vi "KH7008 Parse Response String.vi"(8 "error in (no error)":errorcluster, 11 "Response String":string) -> (0 "error out":errorcluster, 3 "Channel Parameters":T1)   [LabVIEW 2019, in "Inst.Krohn-Hite-7008.lvclass"]
uses:
  Inst.Krohn-Hite-7008.lvclass
  Typedefs/SetAll-Cluster.ctl
  Typedefs/Channel-Enum.ctl
  Typedefs/Gain-Enum.ctl
  Typedefs/Filter-Enum.ctl
  Typedefs/Shunt-Enum.ctl
  Typedefs/Coupling-Enum.ctl
  Typedefs/Input Configuration-Enum.ctl
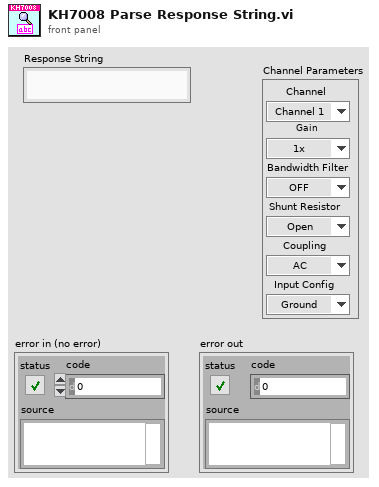
[diagram p1: front panel]
types:
  T1 = typedef "Inst.Krohn-Hite-7008.lvclass/SetAll-Cluster.ctl" = cluster{"Channel":T2, "Gain":T3, "Bandwidth Filter":T4, "Shunt Resistor":T5, "Coupling":T6, "Input Config":T7}
  T2 = typedef "Inst.Krohn-Hite-7008.lvclass/Channel-Enum.ctl" = enum16{"Channel 1", "Channel 2", "Channel 3", "Channel 4", "Channel 5", "Channel 6", "Channel 7", "Channel 8"}
  T3 = typedef "Inst.Krohn-Hite-7008.lvclass/Gain-Enum.ctl" = enum16{"1x", "10x", "100x", "1000x"}
  T4 = typedef "Inst.Krohn-Hite-7008.lvclass/Filter-Enum.ctl" = enum16{"OFF", "ON"}
  T5 = typedef "Inst.Krohn-Hite-7008.lvclass/Shunt-Enum.ctl" = enum16{"Open", "50 Ohms", "500 Ohms", "5k Ohms", "50k Ohms", "10M Ohm"}
  T6 = typedef "Inst.Krohn-Hite-7008.lvclass/Coupling-Enum.ctl" = enum16{"AC", "DC"}
  T7 = typedef "Inst.Krohn-Hite-7008.lvclass/Input Configuration-Enum.ctl" = enum16{"Ground", "SE+ (-gnd)", "SE- (+gnd)", "Differential"}
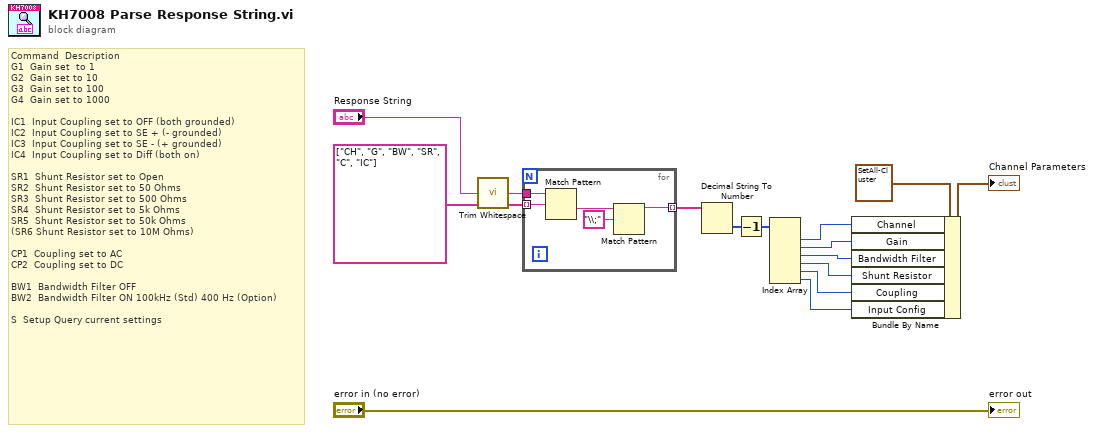
[diagram p0: block diagram]
diagram:
  # "Command  Description \nG1  Gain set  to 1 \nG2  Gain set to 10 \nG3  Gain set to 100 \nG4  Gain set to 1000 \n   \nIC1  Input Coupling set to OFF (both grounded) \nIC2  Input Coupling set to SE + (- grounded) \nIC3  Input Coupling set to SE - (+ grounded) \nIC4  Input Coupling set to Diff (both on) \n   \nSR1  Shunt Resistor set to Open \nSR2  Shunt Resistor set to 50 Ohms \nSR3  Shunt Resistor set to 500 Ohms \nSR4  Shunt Resistor set to 5k Ohms \nSR5  Shunt Resistor set to 50k Ohms \n(SR6 Shunt Resistor set to 10M Ohms)\n   \nCP1  Coupling set to AC \nCP2  Coupling set to DC \n   \nBW1  Bandwidth Filter OFF \nBW2  Bandwidth Filter ON 100kHz (Std) 400 Hz (Option)\n   \nS  Setup Query current settings"
  n1 = call <vilib>:"Trim Whitespace.vi"("string"="Response String") -> ("trimmed string"=w2:string)  [unwired: 1 in]
  n2 = for {
    tunnel: string[] ["CH", "G", "BW", "SR", "C", "IC"] ("operators (none)") -> [w19] mode=indexing
    tunnel: [w16] -> w12 mode=indexing
    tunnel: w2 -> [w17]
    n3 = Match Pattern(string=w17, regular expression=w19) -> (after substring=w20:string)  [unwired: 1 in, 3 out]
    n4 = Match Pattern(string=w20, regular expression="\\;") -> (before substring=w16:string)  [unwired: 1 in, 3 out]
  }
  n5 = Decimal String To Number(string=w12) -> (number=w11:i32[])  [unwired: 2 in, 1 out]
  n6 = Decrement(x=w11) -> (x-1=w10:i32[])
  n7 = Index Array(array=w10) -> (element #1=w9:i32, element #2=w8:i32, element #3=w7:i32, element #4=w6:i32, element #5=w5:i32, element #6=w4:i32)  [unwired: 6 in]
  n8 = Bundle By Name(cluster=T1 {"Channel"=enum."Channel 1", "Gain"=enum."1x", "Bandwidth Filter"=enum."OFF", "Shunt Resistor"=enum."Open", "Coupling"=enum."AC", "Input Config"=enum."Ground"} ("Channel Parameters 2"), "Channel"=w9, "Gain"=w8, "Bandwidth Filter"=w7, "Shunt Resistor"=w6, "Coupling"=w5, "Input Config"=w4) -> (→"Channel Parameters":T1)
  "error out" <- "error in (no error)"
